vi "Measurement Logic.vi"() -> ()   [LabVIEW 2020, in "Waveform Measurement.lvlib"]
uses:
  Waveform Measurement.lvlib
  <vilib>/MeasurementLink/MeasurementLink Measurement Server/Measure Call Context/Measure Call Context.lvclass
  Measurement Configuration.ctl
  Measurement Results.ctl
  <vilib>/gRPC/Generated APIs/ni/protobuf/types/RPC Messages/ni_protobuf_types_DoubleAnalogWaveform_Flat.ctl
  <vilib>/gRPC/Generated APIs/ni/protobuf/types/RPC Messages/ni_protobuf_types_PrecisionTimestamp_Flat.ctl
  <vilib>/gRPC/Generated APIs/ni/protobuf/types/RPC Messages/ni_protobuf_types_DoubleAnalogWaveform_AttributesEntry_Flat.ctl
  <vilib>/gRPC/Generated APIs/ni/protobuf/types/RPC Messages/ni_protobuf_types_WaveformAttributeValue_Flat.ctl
  <vilib>/gRPC/Generated APIs/ni/protobuf/types/ni.protobuf.types.lvlib
  <vilib>/measure/NI_MABase.lvlib
  <vilib>/gRPC/Extensions/Extensions.lvlib
panel:
  out "measurement results":T1
  in  "measurement configuration":T6={"Signal Type"=enum."Sine", "Number of Samples"=1000, "Amplitude"=1.0, "Frequency"=10.0, "Sample Rate"=1000, "Offset"=0.0}
  out "measure call context out":refnum<class "Measure Call Context.lvclass">
  in  "measure call context in":refnum<class "Measure Call Context.lvclass">
  out "error out":errorcluster
  in  "error in":errorcluster
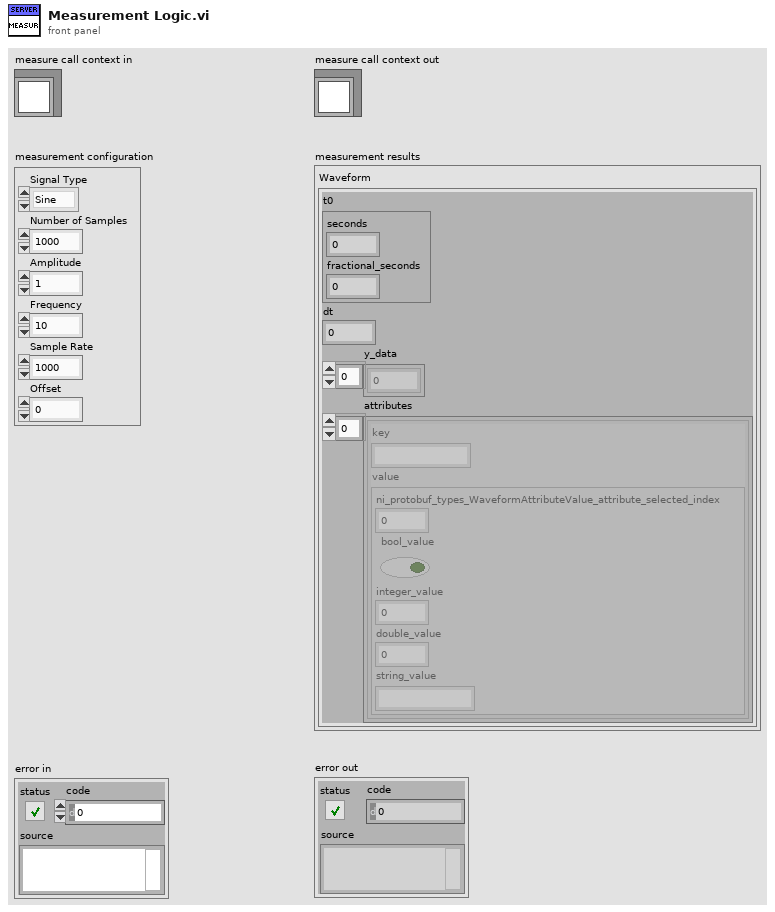
[diagram p1: front panel]
types:
  T1 = typedef "Waveform Measurement.lvlib/Measurement Results.ctl" = cluster{"Waveform":T2}
  T2 = typedef "ni.protobuf.types.lvlib/ni_protobuf_types_DoubleAnalogWaveform_Flat.ctl" = cluster{"t0":T3, "dt":dbl, "y_data":dbl[], "attributes":T4[]}
  T3 = typedef "ni.protobuf.types.lvlib/ni_protobuf_types_PrecisionTimestamp_Flat.ctl" = cluster{"seconds":i64, "fractional_seconds":u64}
  T4 = typedef "ni.protobuf.types.lvlib/ni_protobuf_types_DoubleAnalogWaveform_AttributesEntry_Flat.ctl" = cluster{"key":string, "value":T5}
  T5 = typedef "ni.protobuf.types.lvlib/ni_protobuf_types_WaveformAttributeValue_Flat.ctl" = cluster{"ni_protobuf_types_WaveformAttributeValue_attribute_selected_index":i32, "bool_value":bool, "integer_value":i32, "double_value":dbl, "string_value":string}
  T6 = typedef "Waveform Measurement.lvlib/Measurement Configuration.ctl" = cluster{"Signal Type":enum32{"None", "Sine", "Square", "Triangle", "Sawtooth"}, "Number of Samples":u32, "Amplitude":dbl, "Frequency":dbl, "Sample Rate":u32, "Offset":dbl}
  T7 = enum32{"None", "Sine", "Square", "Triangle", "Sawtooth"}
  T8 = cluster{"Sample Rate":u32, "Number of Samples":u32}
  T9 = enum16{"Sine Wave", "Triangle Wave", "Square Wave", "Sawtooth Wave"}
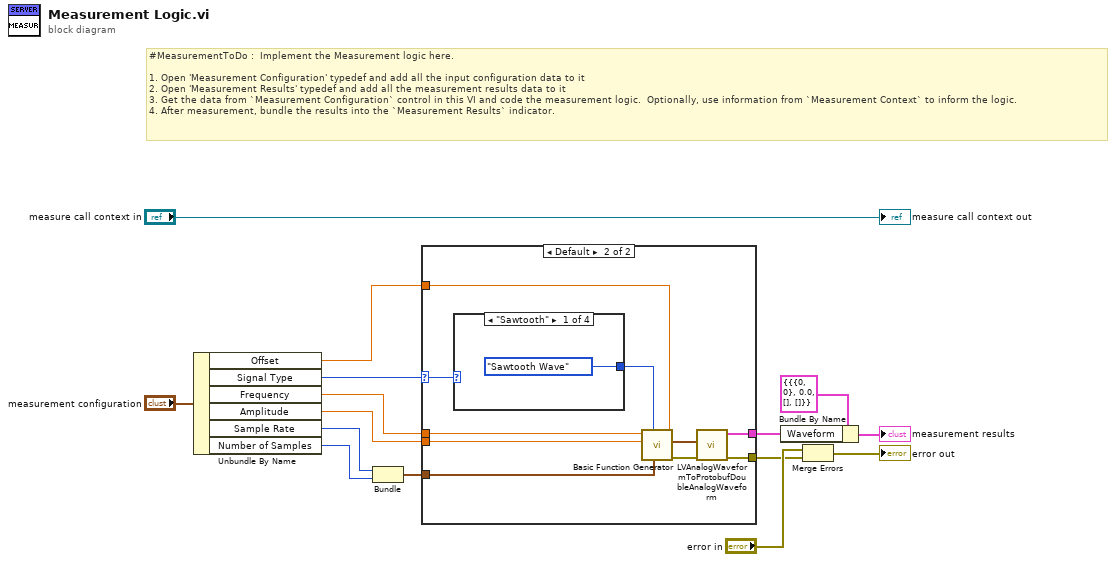
[diagram p0: block diagram]
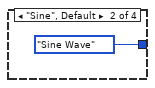
[diagram p3: hidden frame]
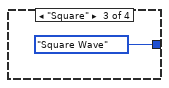
[diagram p4: hidden frame]
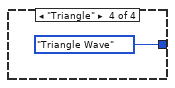
[diagram p5: hidden frame]
diagram:
  # "#MeasurementToDo :  Implement the Measurement logic here.\n\n1. Open 'Measurement Configuration' typedef and add all the input configuration data to it\n2. Open 'Measurement Results' typedef and add all the measurement results data to it\n3. Get the data from `Measurement Configuration` control in this VI and code the measurement logic.  Optionally, use information from `Measurement Context` to inform the logic.\n4. After measurement, bundle the results into the `Measurement Results` indicator."
  n1 = Unbundle By Name("measurement configuration") -> ("Offset"=w13:dbl, "Signal Type"=w7:T7, "Frequency"=w12:dbl, "Amplitude"=w11:dbl, "Sample Rate"=w10:u32, "Number of Samples"=w9:u32)
  n2 = Bundle("Sample Rate"=w10, "Number of Samples"=w9) -> (w8:T8)  [unwired: 1 in]
  n3 = case shown="Default" w7 {
    selector: w7 -> [_ w25]
    tunnel: w13 -> [_ w23]
    tunnel: w12 -> [_ w22]
    tunnel: w11 -> [_ w21]
    tunnel: w8 -> [_ w20]
    tunnel: [_ w18] -> w6
    tunnel: [_ w16] -> w1
    frame "None" {
    }
    frame Default {
      n4 = case shown="\"Sawtooth\"" w25 {
        tunnel: [T9."Sawtooth Wave" ("signal type") T9."Sine Wave" ("signal type") T9."Square Wave" ("signal type") T9."Triangle Wave" ("signal type")] -> w24
        frame "Sawtooth" {
        }
        frame "Sine", Default {
        }
        frame "Square" {
        }
        frame "Triangle" {
        }
      }
      n5 = call <vilib>:"Basic Function Generator.vi"("offset"=w23, "sampling info"=w20, "signal type"=w24, "amplitude"=w21, "frequency"=w22) -> ("error out"=w17:errorcluster, "signal out"=w19:waveform(dbl))  [unwired: 4 in, 1 out]
      n6 = call <vilib>:"LVAnalogWaveformToProtobufDoubleAnalogWaveform.vi"("error in (no error)"=w17, "Waveform"=w19) -> ("error out"=w16:errorcluster, "ni_protobuf_types_DoubleAnalogWaveform_Flat"=w18:T2)  [unwired: 8 in]
    }
  }
  n7 = Bundle By Name(cluster=T1 {"Waveform"={"t0"={"seconds"=0, "fractional_seconds"=0}, "dt"=0.0, "y_data"=[], "attributes"=[]}} ("Measurement Results"), "Waveform"=w6) -> (→"measurement results":T1)
  n8 = Merge Errors("error in", w1) -> (→"error out":errorcluster)
  "measure call context out" <- "measure call context in"
